vi "check_crc.vi"(1 "Data":u8[](array[numeric])) -> (0 "CRC check":bool)   [LabVIEW 2022 SP3]
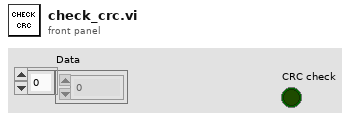
[diagram p1: front panel]
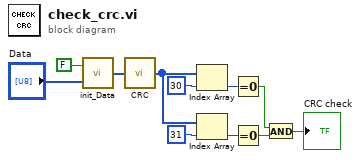
[diagram p0: block diagram]
diagram:
  n1 = call "init_Data.vi"("Input"="Data", "Zerar CRC"=FALSE) -> ("Output"=w9:u8[])
  n2 = call "CRC.vi"("Data"=w9) -> ("Data + CRC"=w7:u8[])
  n3 = Index Array(array=w7, index=30) -> (element=w4:u8)
  n4 = Index Array(array=w7, index=31) -> (element=w3:u8)
  n5 = Equal To 0?(x=w4) -> (x = 0?=w1:bool)
  n6 = Equal To 0?(x=w3) -> (x = 0?=w2:bool)
  n7 = And(x=w1, y=w2) -> (x .and. y?=→"CRC check":bool)
